vi "FilterAirmar.vi"(10 "Notifier":refnum<notifier>, 11 "Queue in":refnum<queue>) -> ()   [LabVIEW 2013]
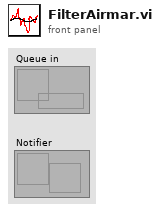
[diagram p1: front panel]
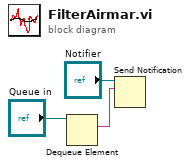
[diagram p0: block diagram]
diagram:
  n1 = Dequeue Element(queue="Queue in") -> (element=w2:string)  [unwired: 2 in, 3 out]
  n2 = Send Notification(notification=w2, notifier="Notifier") -> ()  [unwired: 1 in, 2 out]
